vi "ConstructorContextMenuRTM.vi"(8 "error in (no error)":errorcluster, 9 "RTM Path":path, 10 "CtrlRef":refnum<vi>, 11 "Menu in":refnum<class "Menu.lvclass">) -> (0 "error out":errorcluster, 2 "MenuSelectionEvent":refnum<user-event>, 3 "Menu out":refnum<class "Menu.lvclass">)   [LabVIEW 2021, in "Menu.lvlib" / "Menu.lvclass"]
uses:
  Menu.lvclass
  MenuSelection.ctl
  Menu.lvclass/Menu.ctl
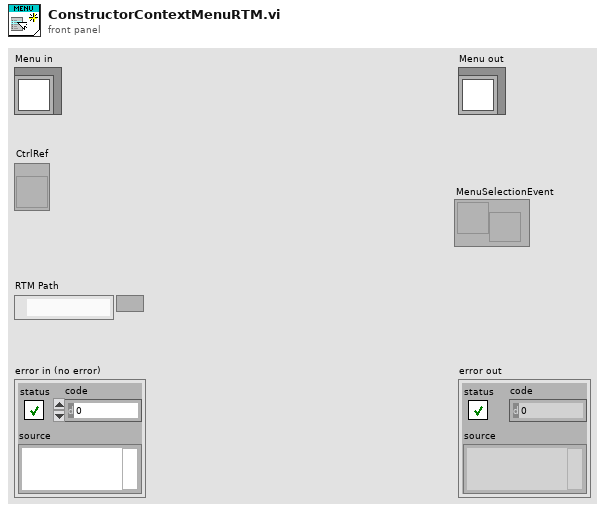
[diagram p1: front panel]
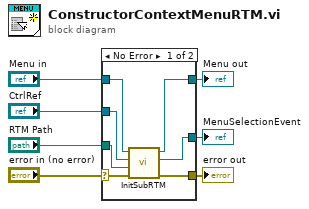
[diagram p0: block diagram]
diagram:
  n1 = case shown="No Error" "error in (no error)" {
    selector: "error in (no error)" -> [w13 w16]
    tunnel: [w11 w16] -> w6
    tunnel: [w12 w15] -> w4
    tunnel: "Menu in" -> [w14 w15]
    tunnel: "CtrlRef" -> [w8 _]
    tunnel: [w10 _] -> w2
    tunnel: "RTM Path" -> [w9 _]
    frame No Error {
      n2 = call "InitSubRTM.vi"("error in (no error)"=w13, "RTM Path"=w9, "CtrlRef"=w8, "Menu in"=w14) -> ("error out"=w11:errorcluster, "MenuSelectionEvent"=w10:refnum<user-event>, "Menu out"=w12:refnum<class "Menu.lvclass">)  [unwired: 5 in]
    }
    frame Error {
    }
  }
  "error out" <- w6
  "Menu out" <- w4
  "MenuSelectionEvent" <- w2
